vi "WPI_MXP PWM Channel to MXP Pin.vi"(7 "PWMChannel":T1) -> (8 "Shared MXP Pin":T2)   [LabVIEW 2017]
uses:
  <vilib>/Rock Robotics/WPI/MXP/WPI_MXP Shared MXP Pin.ctl
  <vilib>/Rock Robotics/SystemInterfaces/DIO/FPGA_DIOPWMChannel.ctl
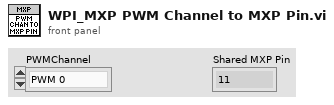
[diagram p1: front panel]
types:
  T1 = typedef "FPGA_DIOPWMChannel.ctl" = enum8{"PWM 0", "PWM 1", "PWM 2", "PWM 3", "PWM 4", "PWM 5", "PWM 6", "PWM 7", "PWM 8", "PWM 9", "PWM MXP 0", "PWM MXP 1", "PWM MXP 2", "PWM MXP 3", "PWM MXP 4", "PWM MXP 5", "PWM MXP 6", "PWM MXP 7", "PWM MXP 8", "PWM MXP 9", "Invalid"}
  T2 = typedef "WPI_MXP Shared MXP Pin.ctl" = enum16{"11", "13", "15", "17", "19", "21", "23", "25", "27", "29", "31", "18", "22", "26", "32", "34", "Invalid"}
  T3 = enum16{"11", "13", "15", "17", "19", "21", "23", "25", "27", "29", "31", "18", "22", "26", "32", "34", "Invalid"}
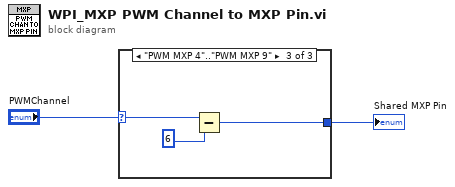
[diagram p0: block diagram]
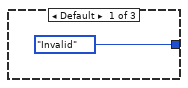
[diagram p2: hidden frame]
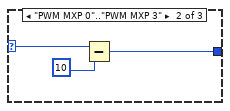
[diagram p3: hidden frame]
diagram:
  n1 = case shown="\"PWM MXP 4\"..\"PWM MXP 9\"" "PWMChannel" {
    selector: "PWMChannel" -> [_ w6 w9]
    tunnel: [T3."Invalid" ("Shared MXP Pin") w4 w7] -> w1
    frame Default {
    }
    frame "PWM MXP 0".."PWM MXP 3" {
      n2 = Subtract(x=w6, y=u8 10) -> (x-y=w4:u8)
    }
    frame "PWM MXP 4".."PWM MXP 9" {
      n3 = Subtract(x=w9, y=u8 6) -> (x-y=w7:u8)
    }
  }
  "Shared MXP Pin" <- w1
